vi "New_System.vi"() -> ()   [LabVIEW 2023]
uses:
  <vilib>/Modbus/master/Modbus Master.lvclass
  <vilib>/NI/Modbus Library/API/Master/Modbus Master.lvclass
  <vilib>/Modbus/master/Create Master Instance (TCP).vi
panel:
  in  "Slide":dbl(slide) scale=0.0..10.0
  in  "Tab Control":T1(tab)
  out "Run Status":bool
  out "Stop Status":bool
  in  "Run":bool
  out "Lower Limit":bool
  in  "Lower Limit":dbl
  out "Lvl 2":dbl
  out "Lvl 2":bool
  out "Lvl 3":dbl
  out "Lvl 3":bool
  out "Lvl 4":dbl
  out "Lvl 4":bool
  out "Alarm":bool
  in  "Upper Limit":dbl
  out "Machine Current Temp (°C)":dbl
  out "Machine Temp Thermometer":dbl(slide) scale=0.0..100.0
  in  "Stop":bool
  out "Fan Speed":dbl(knob) scale=0.0..5.0
  out "Total Actuations":u16
  out "Fails":u16
  out "Passes":u16
  out "Status":u16
  out "Sealer Status":bool
  out "Off":bool
  out "On":bool
  in  "Slave IP Address":string
  in  "stop":bool
  out "Change Plunger":bool
  # "Soft Drink Production Monitering System"
  # "Machine's Temperature (°C)"
  # "Critical Temperature Levels"
  # "Please enter upper & lower limits."
  # "Upper Limit"
  # "Level 4"
  # "Level 3"
  # "Level 2"
  # "Lower Limit"
  # "RUN"
  # "STOP"
  # "Power"
  # "Machine Status"
  # "Modbus Master"
  # "Please enter relevant address."
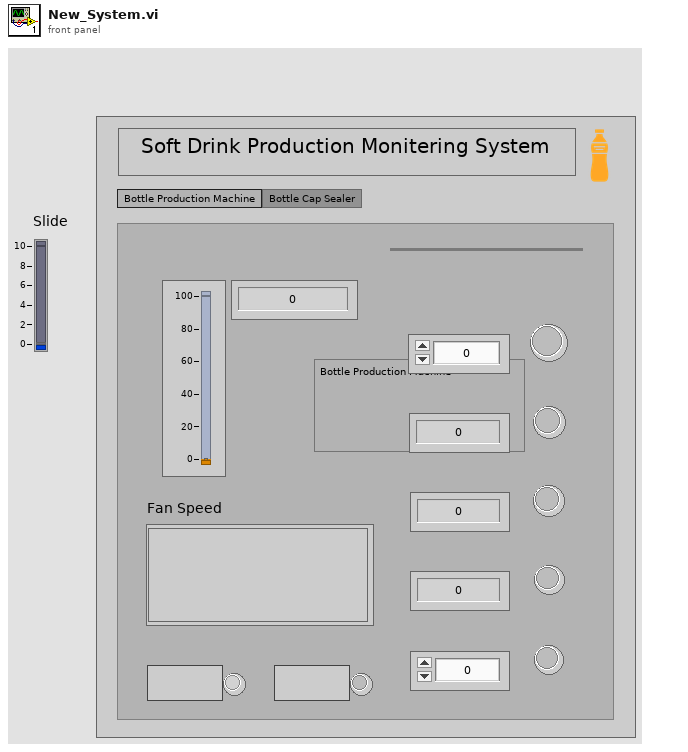
[diagram p1: front panel]
types:
  T1 = enum32{"Bottle Production Machine", "Bottle Cap Sealer"}
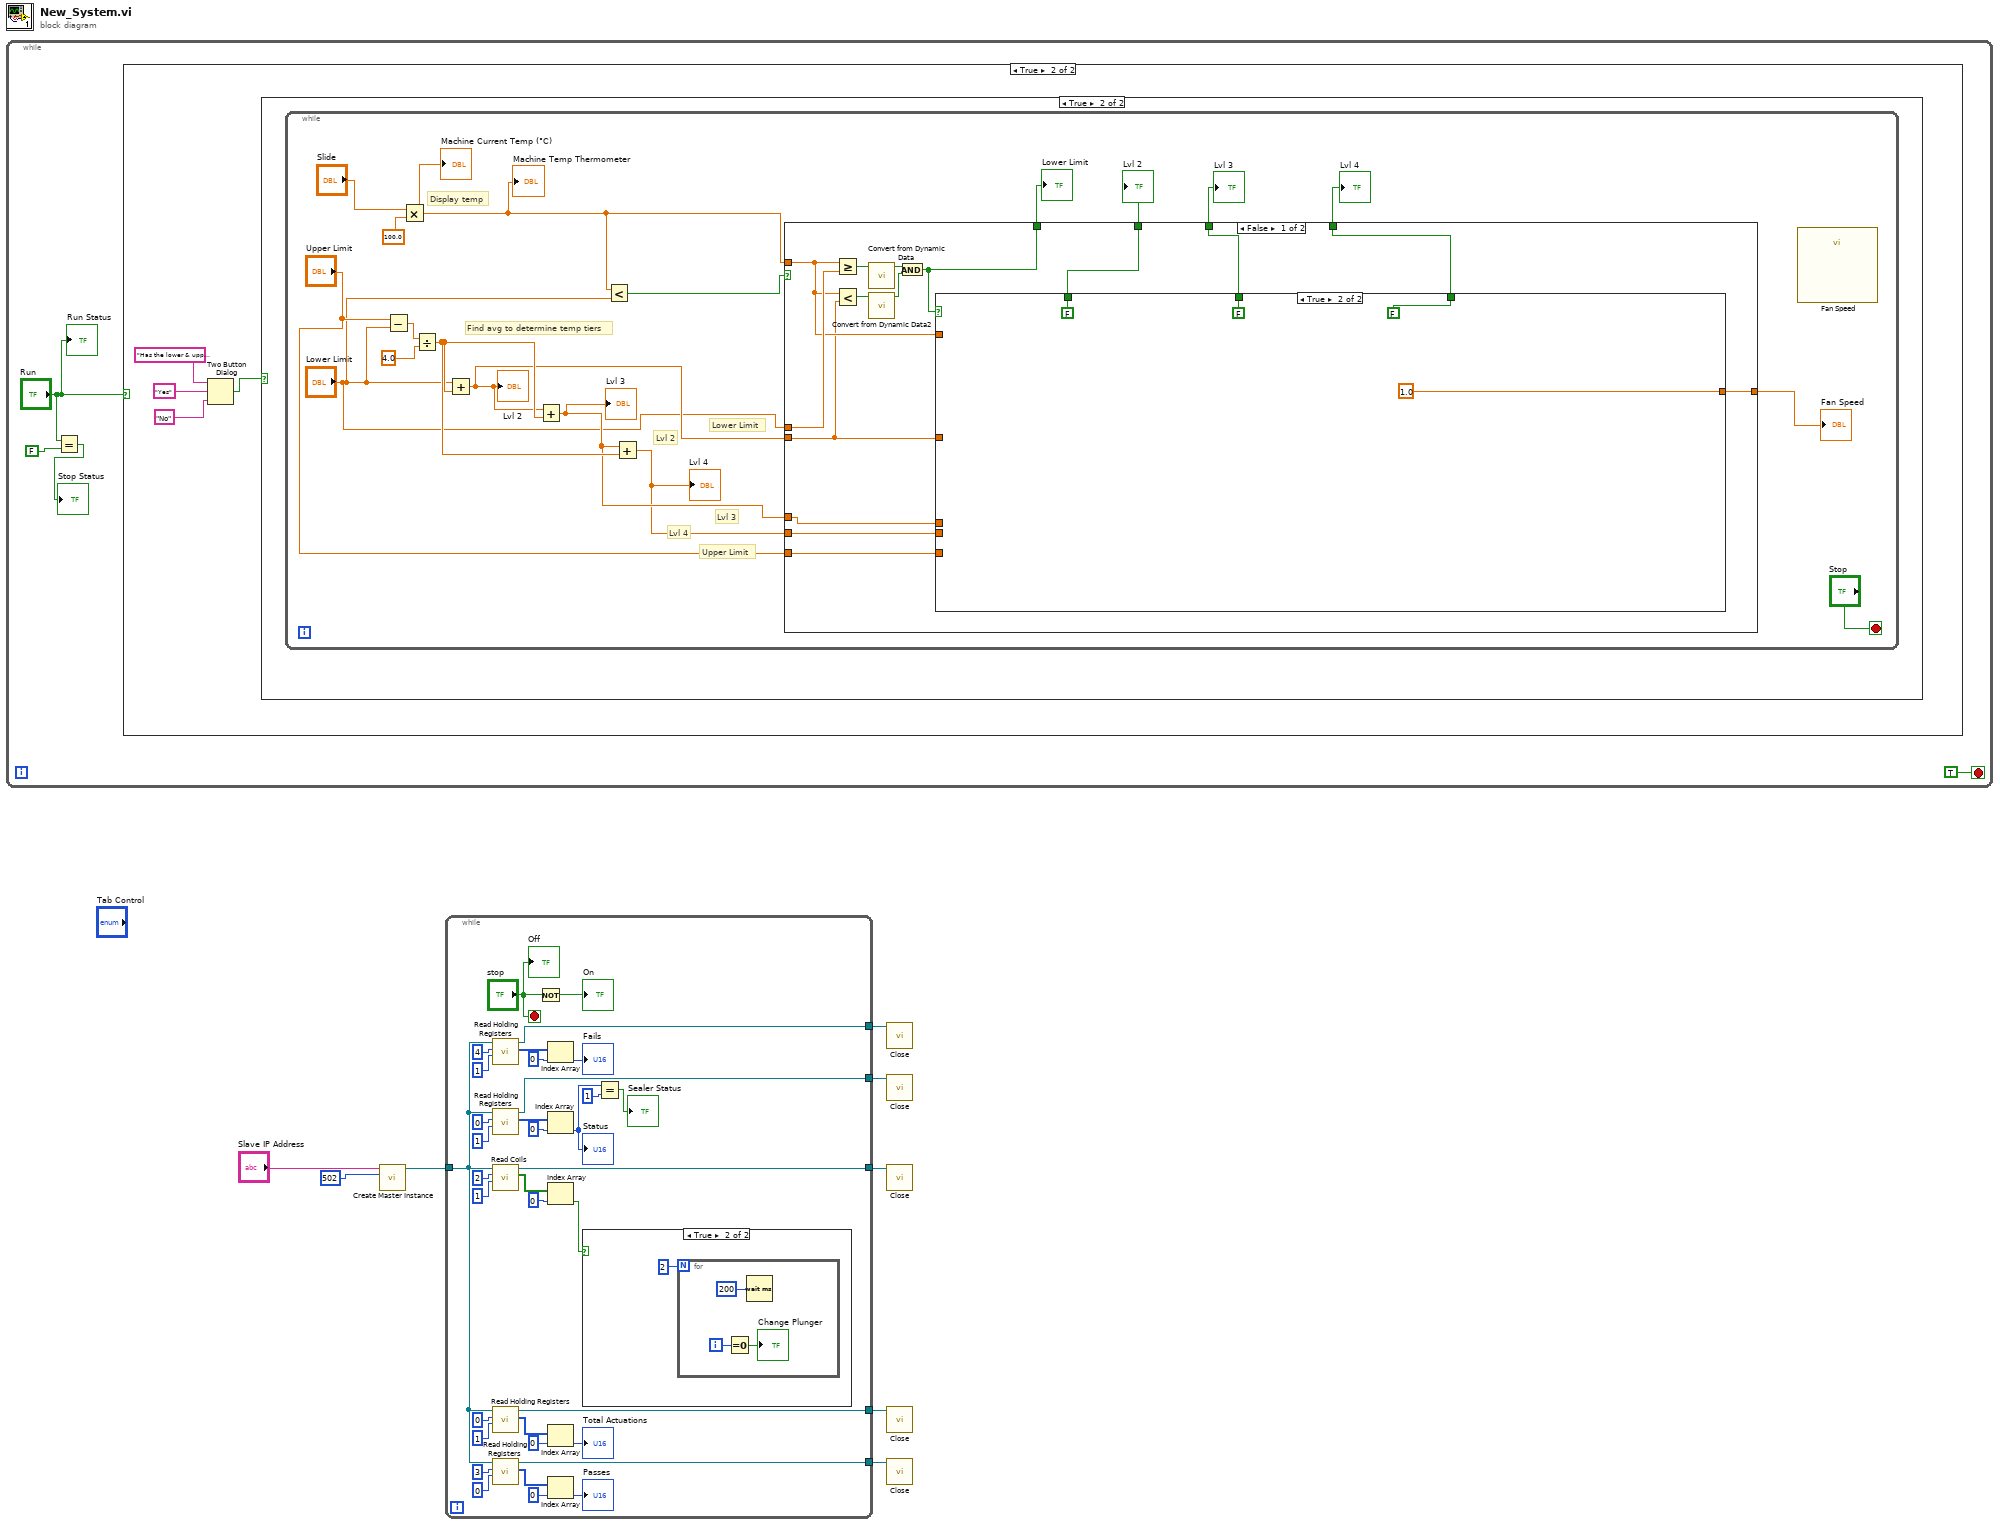
[diagram p0: block diagram]
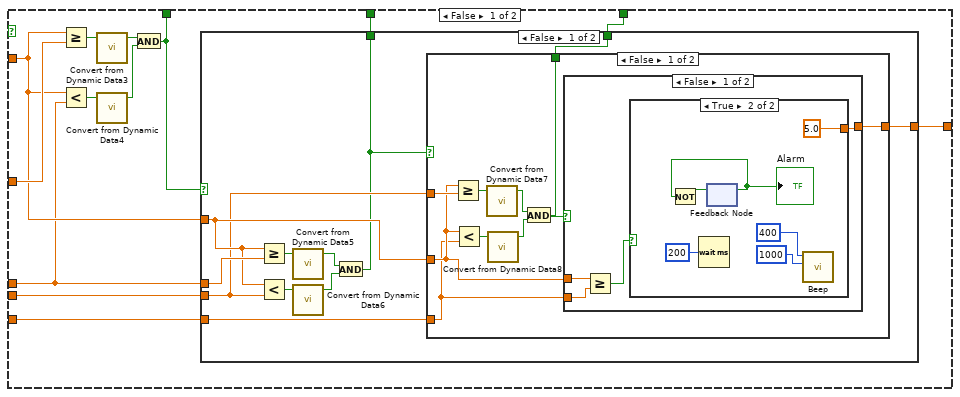
[diagram p4: hidden frame]
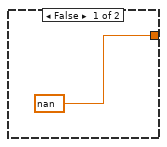
[diagram p5: hidden frame]
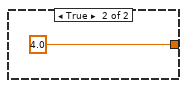
[diagram p6: hidden frame]
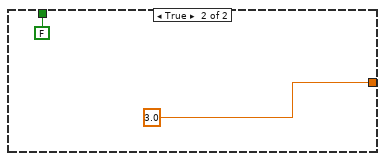
[diagram p7: hidden frame]
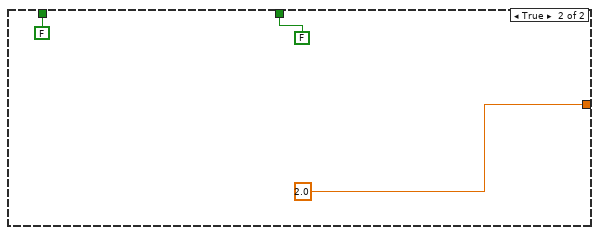
[diagram p8: hidden frame]
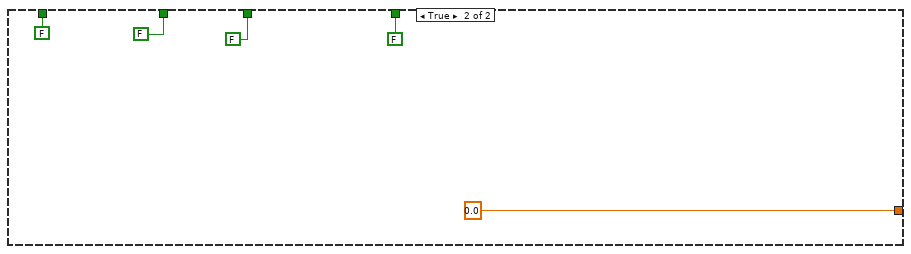
[diagram p9: hidden frame]
diagram:
  n1 = while {
    stop <- TRUE stop-if-true
    n2 = Equal?(x="Run", y=FALSE) -> (x = y?=→"Stop Status":bool)
    n3 = case shown="True" "Run" {
      frame False {
      }
      frame True {
        n4 = Two Button Dialog(message="Has the lower & upper limit been entered?", 1:"No" ("F button name (\"Cancel\")"), 2:"Yes" ("T button name (\"OK\")")) -> (T button?=w13:bool)
        n5 = case shown="True" w13 {
          frame False {
          }
          frame True {
            n6 = while {
              stop <- "Stop" stop-if-true
              # "Display temp"
              # "Lvl 4"
              # "Lvl 3"
              # "Upper Limit"
              # "Lvl 2"
              # "Lower Limit"
              # "Find avg to determine temp tiers"
              n7 = Subtract(x="Upper Limit", y="Lower Limit") -> (x-y=w34:dbl)
              n8 = Multiply(x="Slide", y=100.0) -> (x*y=w19:dbl)
              "Machine Temp Thermometer" <- w19
              "Machine Current Temp (°C)" <- w19
              n9 = Divide(x=w34, y=4.0) -> (x/y=w32:dbl)
              n10 = Add(x="Lower Limit", y=w32) -> (x+y=w28:dbl)
              "Lvl 2" <- w28
              n11 = Add(x=w28, y=w32) -> (x+y=w27:dbl)
              "Lvl 3" <- w27
              n12 = Less?(x=w19, y="Lower Limit") -> (x < y?=w30:bool)
              n13 = Add(x=w27, y=w32) -> (x+y=w26:dbl)
              "Lvl 4" <- w26
              n14 = case shown="False" w30 {
                tunnel: [w48 0.0 ("y")] -> w29
                tunnel: w19 -> [w47 _]
                tunnel: "Lower Limit" -> [w49 _]
                tunnel: w28 -> [w44 _]
                tunnel: w27 -> [w43 _]
                tunnel: w26 -> [w45 _]
                tunnel: "Upper Limit" -> [w46 _]
                tunnel: [w38 FALSE] -> w25
                tunnel: [w37 FALSE] -> w24
                tunnel: [w36 FALSE] -> w23
                tunnel: [w35 FALSE] -> w22
                frame False {
                  n15 = Greater Or Equal?(x=w47, y=w49) -> (x >= y?=w42:bool)
                  n16 = Less?(x=w47, y=w44) -> (x < y?=w41:bool)
                  n17 = call "Convert from Dynamic Data"("Dynamic Data Type"=w42) -> ("Scalar"=w40:bool)  [unwired: 3 in]
                  n18 = call "Convert from Dynamic Data2"("Dynamic Data Type"=w41) -> ("Scalar"=w39:bool)  [unwired: 3 in]
                  n19 = And(x=w40, y=w39) -> (x .and. y?=w38:bool)
                  n20 = case shown="True" w38 {
                    tunnel: [w61 1.0 ("y")] -> w48
                    tunnel: w44 -> [w62 _]
                    tunnel: w43 -> [w58 _]
                    tunnel: w47 -> [w59 _]
                    tunnel: w45 -> [w57 _]
                    tunnel: w46 -> [w60 _]
                    tunnel: [w52 FALSE] -> w37
                    tunnel: [w51 FALSE] -> w36
                    tunnel: [w50 FALSE] -> w35
                    frame False {
                      n21 = Greater Or Equal?(x=w59, y=w62) -> (x >= y?=w56:bool)
                      n22 = Less?(x=w59, y=w58) -> (x < y?=w55:bool)
                      n23 = call "Convert from Dynamic Data3"("Dynamic Data Type"=w56) -> ("Scalar"=w54:bool)  [unwired: 3 in]
                      n24 = call "Convert from Dynamic Data4"("Dynamic Data Type"=w55) -> ("Scalar"=w53:bool)  [unwired: 3 in]
                      n25 = And(x=w54, y=w53) -> (x .and. y?=w52:bool)
                      n26 = case shown="False" w52 {
                        tunnel: [w72 2.0 ("y")] -> w61
                        tunnel: w59 -> [w71 _]
                        tunnel: w58 -> [w73 _]
                        tunnel: w57 -> [w69 _]
                        tunnel: w60 -> [w70 _]
                        tunnel: [w64 FALSE] -> w51
                        tunnel: [w63 FALSE] -> w50
                        frame False {
                          n27 = Greater Or Equal?(x=w71, y=w73) -> (x >= y?=w68:bool)
                          n28 = Less?(x=w71, y=w69) -> (x < y?=w67:bool)
                          n29 = call "Convert from Dynamic Data5"("Dynamic Data Type"=w68) -> ("Scalar"=w66:bool)  [unwired: 3 in]
                          n30 = call "Convert from Dynamic Data6"("Dynamic Data Type"=w67) -> ("Scalar"=w65:bool)  [unwired: 3 in]
                          n31 = And(x=w66, y=w65) -> (x .and. y?=w64:bool)
                          n32 = case shown="False" w64 {
                            tunnel: [w81 3.0 ("y")] -> w72
                            tunnel: w69 -> [w82 _]
                            tunnel: w71 -> [w76 _]
                            tunnel: w70 -> [w75 _]
                            tunnel: [w74 FALSE] -> w63
                            frame False {
                              n33 = Greater Or Equal?(x=w76, y=w82) -> (x >= y?=w80:bool)
                              n34 = Less?(x=w76, y=w75) -> (x < y?=w79:bool)
                              n35 = call "Convert from Dynamic Data7"("Dynamic Data Type"=w80) -> ("Scalar"=w78:bool)  [unwired: 3 in]
                              n36 = call "Convert from Dynamic Data8"("Dynamic Data Type"=w79) -> ("Scalar"=w77:bool)  [unwired: 3 in]
                              n37 = And(x=w78, y=w77) -> (x .and. y?=w74:bool)
                              n38 = case shown="False" w74 {
                                tunnel: [w83 4.0 ("y")] -> w81
                                tunnel: w76 -> [w86 _]
                                tunnel: w75 -> [w85 _]
                                frame False {
                                n39 = Greater Or Equal?(x=w86, y=w85) -> (x >= y?=w84:bool)
                                n40 = case shown="True" w84 {
                                tunnel: [nan ("y") 5.0 ("y")] -> w83
                                frame False {
                                }
                                frame True {
                                n41 = Wait (ms)(milliseconds to wait=u32 200) -> ()  [unwired: 1 out]
                                n42 = feedback #1() -> (w88:bool)  [unwired: 1 in]
                                "Alarm" <- w88
                                n43 = Not(x=w88) -> (.not. x?=w90:bool)
                                n44 = feedback-in #1(w90) -> ()
                                n45 = call <vilib>:"Beep.vi"("duration (msec)"=u32 1000, "frequency (Hz)"=u32 400) -> ()  [unwired: 10 in]
                                }
                                }
                                }
                                frame True {
                                }
                              }
                            }
                            frame True {
                            }
                          }
                        }
                        frame True {
                        }
                      }
                    }
                    frame True {
                    }
                  }
                }
                frame True {
                }
              }
              "Fan Speed" <- w29
              "Lower Limit" <- w25
              "Lvl 2" <- w24
              "Lvl 3" <- w23
              "Lvl 4" <- w22
              n46 = call "Fan Speed"() -> ()  [unwired: 18 in, 2 out]
            }
          }
        }
      }
    }
    "Run Status" <- "Run"
  }
  n47 = call-poly <vilib>:"Create Master Instance.vi"("port (502)"=u16 502, "address"="Slave IP Address") -> ("TCP master instance"=w6:refnum<class "Modbus Master.lvclass">)  [unwired: 8 in, 1 out]
  n48 = while {
    tunnel: w6 -> [w128]
    tunnel: [w141] -> w5
    tunnel: [w140] -> w4
    tunnel: [w134] -> w3
    tunnel: [w129] -> w2
    tunnel: [w125] -> w1
    stop <- "stop" stop-if-true
    n49 = call-dynamic "Read Holding Registers.vi"("number of inputs"=u16 1 ("number of holding registers"), "starting address"=u16 4, "Modbus master in"=w128) -> ("register values"=w111:u16[], "Modbus master out"=w125:refnum<class "Modbus Master.lvclass">)  [unwired: 6 in, 1 out]
    n50 = call-dynamic "Read Holding Registers.vi"("number of inputs"=u16 1 ("number of holding registers"), "starting address"=u16 0, "Modbus master in"=w128) -> ("register values"=w118:u16[], "Modbus master out"=w134:refnum<class "Modbus Master.lvclass">)  [unwired: 6 in, 1 out]
    n51 = call-dynamic "Read Coils.vi"("number of inputs"=u16 1 ("number of coils"), "starting address"=u16 2, "Modbus master in"=w128) -> ("coils"=w115:bool[], "Modbus master out"=w141:refnum<class "Modbus Master.lvclass">)  [unwired: 6 in, 1 out]
    n52 = call-dynamic "Read Holding Registers.vi"("number of inputs"=u16 1 ("number of holding registers"), "starting address"=u16 0, "Modbus master in"=w128) -> ("register values"=w121:u16[], "Modbus master out"=w140:refnum<class "Modbus Master.lvclass">)  [unwired: 6 in, 1 out]
    n53 = call-dynamic "Read Holding Registers.vi"("number of inputs"=u16 0 ("number of holding registers"), "starting address"=u16 3, "Modbus master in"=w128) -> ("register values"=w124:u16[], "Modbus master out"=w129:refnum<class "Modbus Master.lvclass">)  [unwired: 6 in, 1 out]
    n54 = Not(x="stop") -> (.not. x?=→"On":bool)
    n55 = Index Array(array=w111, index=0) -> (element=→"Fails":u16)
    n56 = Index Array(array=w118, index=0) -> (element=w116:u16)
    "Status" <- w116
    n57 = Index Array(array=w115, index=0) -> (element=w113:bool)
    n58 = Index Array(array=w121, index=0) -> (element=→"Total Actuations":u16)
    n59 = Index Array(array=w124, index=0) -> (element=→"Passes":u16)
    n60 = case shown="True" w113 {
      frame False {
      }
      frame True {
        n61 = for {
          N: 2 -> [_]
          i -> [w147]
          n62 = Equal To 0?(x=w147) -> (x = 0?=→"Change Plunger":bool)
          n63 = Wait (ms)(milliseconds to wait=u32 200) -> ()  [unwired: 1 out]
        }
      }
    }
    n64 = Equal?(x=w116, y=u16 1 ("number of coils")) -> (x = y?=→"Sealer Status":bool)
    "Off" <- "stop"
  }
  n65 = call-dynamic "Close.vi"("Modbus master in"=w1) -> ()  [unwired: 10 in, 1 out]
  n66 = call-dynamic "Close.vi"("Modbus master in"=w3) -> ()  [unwired: 10 in, 1 out]
  n67 = call-dynamic "Close.vi"("Modbus master in"=w5) -> ()  [unwired: 10 in, 1 out]
  n68 = call-dynamic "Close.vi"("Modbus master in"=w4) -> ()  [unwired: 10 in, 1 out]
  n69 = call-dynamic "Close.vi"("Modbus master in"=w2) -> ()  [unwired: 10 in, 1 out]
